vi "Win32 Window Handle Wrapper.vi"(8 "error in (no error)":errorcluster, 11 "Win32 Window Handle":i32) -> (0 "error out":errorcluster, 3 "System.Windows.Forms.IWin32Window":refnum<k24>)   [LabVIEW 2021]
doc: "This VI Creates a IWin32Window Typed reference a the Win32 Windows Handle.\n\n<b>REFERENCE</b> : https://forums.ni.com/t5/LabVIEW/Make-NET-called-Print-Dialog-frontmost/td-p/219217"
uses:
  System.Windows.Forms
  C:/Development/tsc-material-theme/_Material Theme SubVIs/WindowWrapper.dll
  WindowWrapper.dll
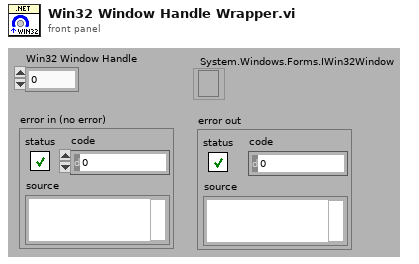
[diagram p1: front panel]
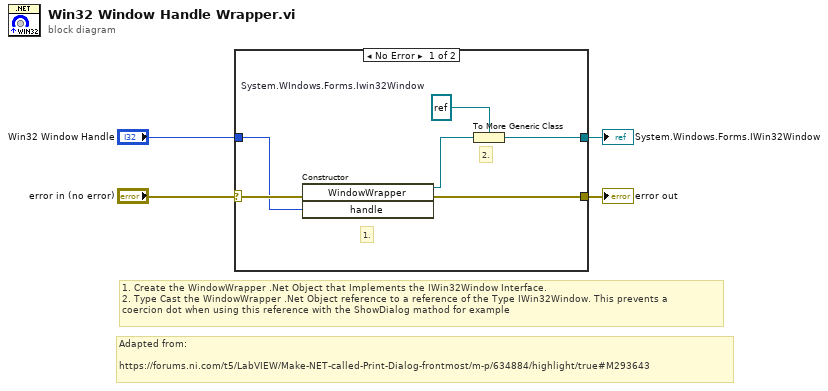
[diagram p0: block diagram]
diagram:
  # "Adapted from:\n\nhttps://forums.ni.com/t5/LabVIEW/Make-NET-called-Print-Dialog-frontmost/m-p/634884/highlight/true#M293643"
  # "1. Create the WindowWrapper .Net Object that Implements the IWin32Window Interface.\n2. Type Cast the WindowWrapper .Net Object reference to a reference of the Type IWin32Window. This prevents a \ncoercion dot when using this reference with the ShowDialog mathod for example"
  n1 = case shown="No Error" "error in (no error)" {
    selector: "error in (no error)" -> [w8 w11]
    tunnel: "Win32 Window Handle" -> [w7 _]
    tunnel: [w6 w11] -> w3
    tunnel: [w9 _] -> w2
    frame No Error {
      w10 = refnum<k24> refnum  # System.WIndows.Forms.Iwin32Window
      # "2."
      # "1."
      n2 = constructor class="WindowWrapper"(error in=w8, "handle"=w7) -> (reference out=w5:refnum<k24>, error out=w6:errorcluster)  [unwired: 2 in, 2 out]
      n3 = To More Generic Class(target class=w10, reference=w5) -> (generic class reference=w9:refnum<k24>)
    }
    frame Error {
    }
  }
  "System.Windows.Forms.IWin32Window" <- w2
  "error out" <- w3
